vi "Raycaster_CalcSpriteScreenX.vi"(10 "Sprite Screen X":i16, 11 "Object Width":i16) -> (3 "Width Calcs":T1)   [LabVIEW 2020]
uses:
  Controls/Raycaster_ScreenCalcs.ctl
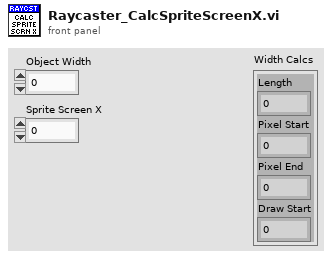
[diagram p1: front panel]
types:
  T1 = typedef "Raycaster_ScreenCalcs.ctl" = cluster{"Length":i16, "Pixel Start":i16, "Pixel End":i16, "Draw Start":i16}
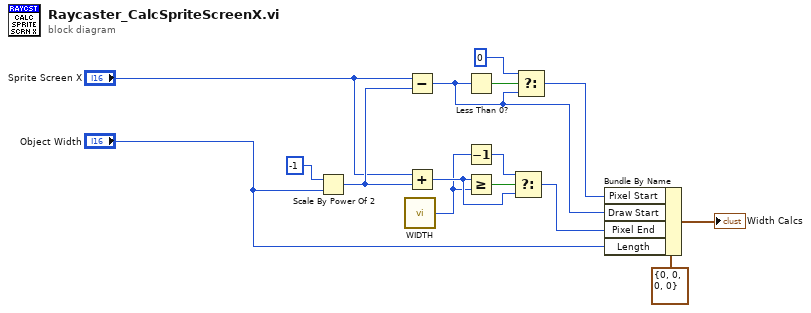
[diagram p0: block diagram]
diagram:
  n1 = Scale By Power Of 2(n=i16 -1, x="Object Width") -> (x*2^n=w5:i16)
  n2 = call "WIDTH.vi"() -> ("WIDTH"=w4:i16)
  n3 = Subtract(x="Sprite Screen X", y=w5) -> (x-y=w1:i16)
  n4 = Add(x="Sprite Screen X", y=w5) -> (x+y=w9:i16)
  n5 = Less Than 0?(x=w1) -> (x < 0?=w14:bool)
  n6 = Decrement(x=w4) -> (x-1=w10:i16)
  n7 = Greater Or Equal?(x=w9, y=w4) -> (x >= y?=w11:bool)
  n8 = Select(t=w10, s=w11, f=w9) -> (s? t:f=w6:i16)
  n9 = Select(t=i16 0, s=w14, f=w1) -> (s? t:f=w7:i16)
  n10 = Bundle By Name(cluster=T1 {"Length"=0, "Pixel Start"=0, "Pixel End"=0, "Draw Start"=0} ("Column Calcs"), "Pixel Start"=w7, "Draw Start"=w1, "Pixel End"=w6, "Length"="Object Width") -> (→"Width Calcs":T1)
